vi "linkam.main.vi"() -> ()   [LabVIEW 8.6]
panel:
  in  "?":bool
  in  "?":bool
  in  "stop 2":bool
  in  "?":bool
  out "Temperature":dbl(graph)
  in  "LN manual\npump speed":u8(slide)
  in  "LN95 setting\nAuto (on) / Manual (off)":bool
  in  "stop":bool
  out "Temperature reading (deg C)":dbl format="%.2g"
  in  "Rate \n(deg/min)":sgl(slide) scale format="%_3g"
  in  "Temperature setting \n(deg C)":dbl format="%.1p"
  in  "VISA resource name in":refnum<visa-resource-name>
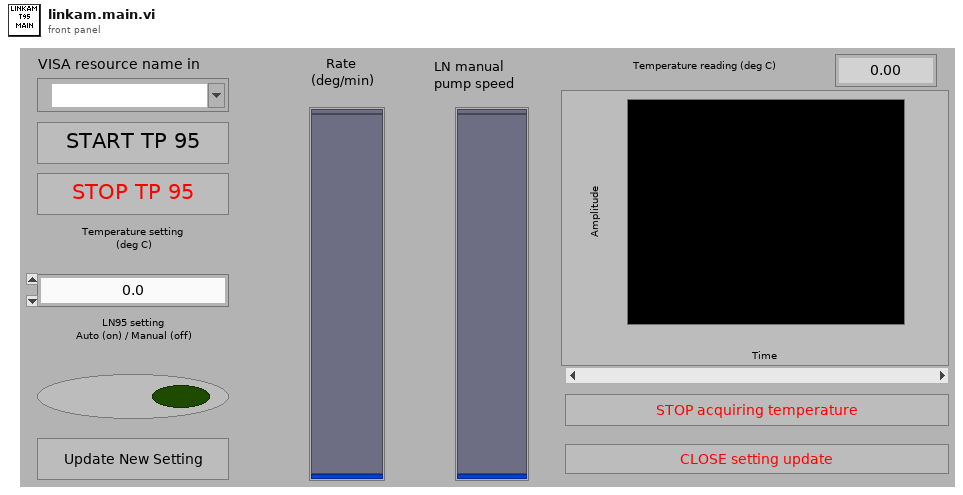
[diagram p1: front panel]
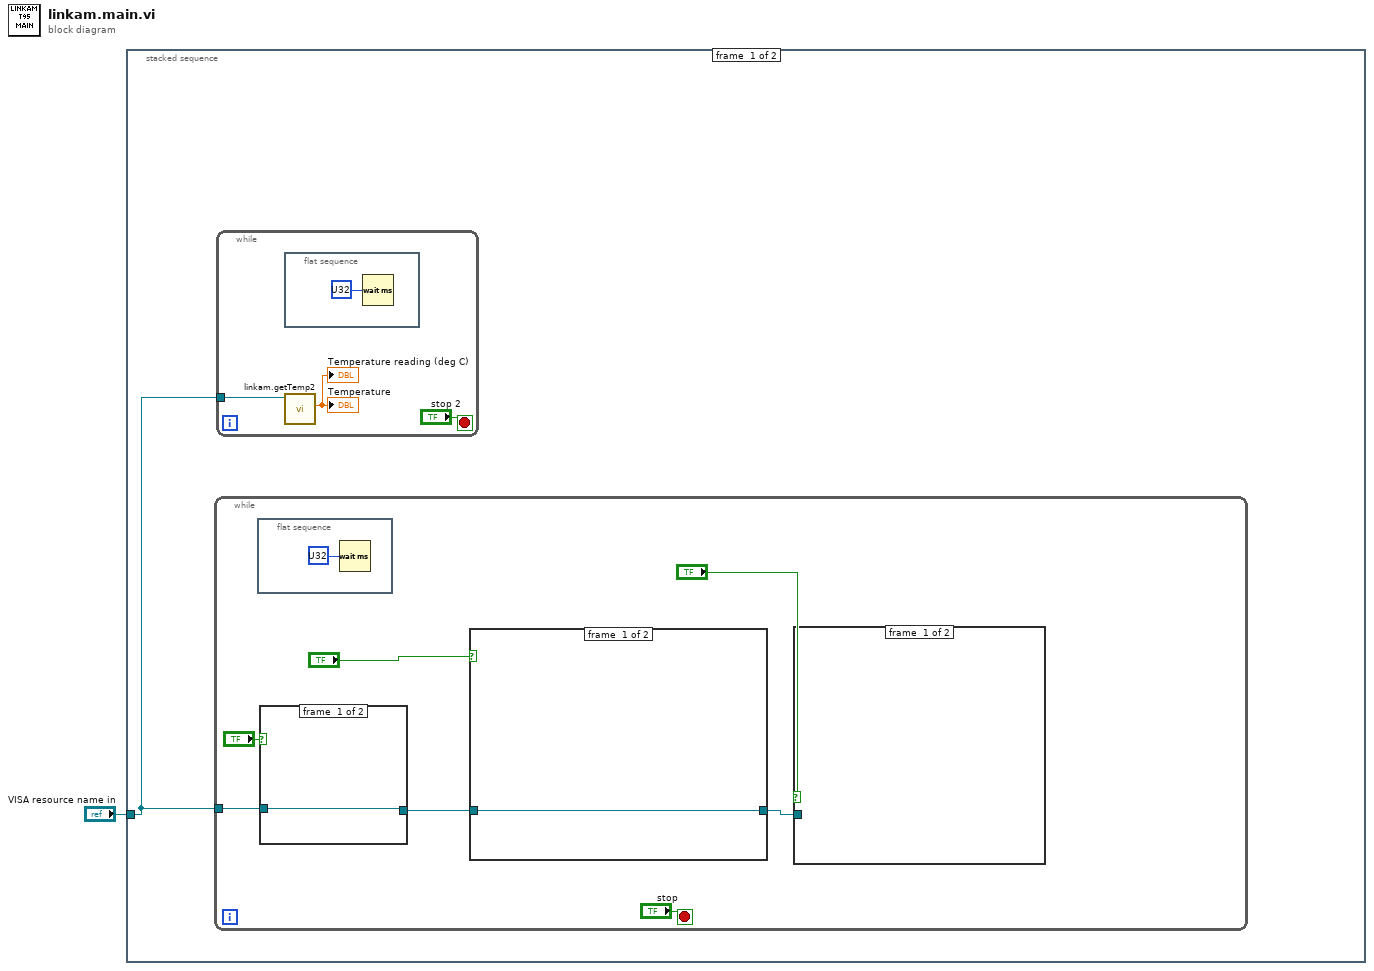
[diagram p0: block diagram]
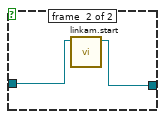
[diagram p2: hidden frame]
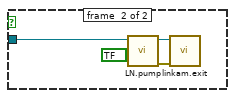
[diagram p3: hidden frame]
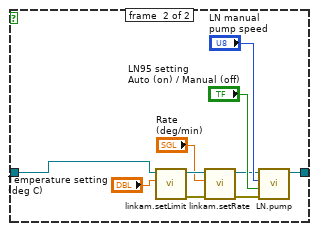
[diagram p4: hidden frame]
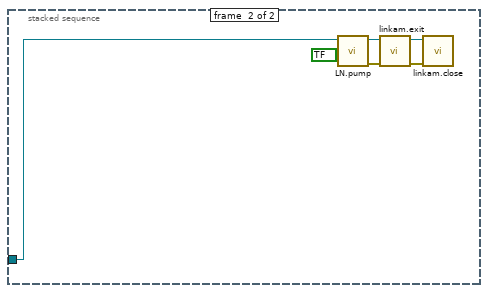
[diagram p5: hidden frame]
diagram:
  n1 = stacked-sequence {
    tunnel: "VISA resource name in" -> [w2 w33]
    frame #0 {
      n2 = while {
        tunnel: w2 -> [w7]
        stop <- "stop" stop-if-true
        n3 = flat-sequence {
          frame #0 {
            n4 = Wait (ms)(milliseconds to wait=u32 ?) -> ()  [unwired: 1 out]
          }
        }
        n5 = case shown="True" "?" {
          tunnel: [w14 w16] -> w9
          tunnel: w7 -> [w14 w15]
          frame #0 {
          }
          frame #1 {
            n6 = call "linkam.start.vi"("VISA resource name in"=w15) -> ("VISA resource name out"=w16:refnum<visa-resource-name>)  [unwired: 9 in, 1 out]
          }
        }
        n7 = case shown="True" "?" {
          tunnel: w9 -> [w21 w23]
          tunnel: [w21 w22] -> w11
          frame #0 {
          }
          frame #1 {
            n8 = call "linkam.setLimit.vi"("temp"="Temperature setting \n(deg C)", "VISA resource name in"=w23) -> ("error out"=w26:errorcluster, "VISA resource name out"=w27:refnum<visa-resource-name>)  [unwired: 8 in]
            n9 = call "linkam.setRate.vi"("error in (no error)"=w26, "rate"="Rate \n(deg/min)", "VISA resource name in"=w27) -> ("error out"=w29:errorcluster, "VISA resource name out"=w28:refnum<visa-resource-name>)  [unwired: 7 in]
            n10 = call "LN.pump.vi"("error in (no error)"=w29, "Auto (on) /Manual (off)"="LN95 setting\nAuto (on) / Manual (off)", "0-30"="LN manual\npump speed", "VISA resource name"=w28) -> ("VISA resource name out"=w22:refnum<visa-resource-name>)  [unwired: 5 in, 1 out]
          }
        }
        n11 = case shown="True" "?" {
          tunnel: w11 -> [_ w17]
          frame #0 {
          }
          frame #1 {
            n12 = call "LN.pump.vi"("Auto (on) /Manual (off)"=bool ?, "VISA resource name"=w17) -> ("error out"=w19:errorcluster, "VISA resource name out"=w20:refnum<visa-resource-name>)  [unwired: 7 in]
            n13 = call "linkam.exit.vi"("error in (no error)"=w19, "VISA resource name in"=w20) -> ()  [unwired: 8 in, 2 out]
          }
        }
      }
      n14 = while {
        tunnel: w2 -> [w3]
        stop <- "stop 2" stop-if-true
        n15 = flat-sequence {
          frame #0 {
            n16 = Wait (ms)(milliseconds to wait=u32 ?) -> ()  [unwired: 1 out]
          }
        }
        n17 = call "linkam.getTemp2.vi"("VISA resource name in"=w3) -> ("temp"=→"Temperature reading (deg C)" →"Temperature":dbl)  [unwired: 8 in, 2 out]
      }
    }
    frame #1 {
      n18 = call "LN.pump.vi"("Auto (on) /Manual (off)"=bool ?, "VISA resource name"=w33) -> ("error out"=w35:errorcluster, "VISA resource name out"=w34:refnum<visa-resource-name>)  [unwired: 7 in]
      n19 = call "linkam.exit.vi"("error in (no error)"=w35, "VISA resource name in"=w34) -> ("error out"=w37:errorcluster, "VISA resource name out"=w38:refnum<visa-resource-name>)  [unwired: 8 in]
      n20 = call "linkam.close.vi"("error in (no error)"=w37, "VISA resource name in"=w38) -> ()  [unwired: 9 in, 1 out]
    }
  }
